vi "Write Data.vi"(8 "error in":errorcluster, 10 "Data":refnum<class "Data.lvclass">, 11 "Update Data MSG in":refnum<class "Update Controller Data MSG.lvclass">) -> (0 "error out":errorcluster, 3 "Update Data MSG out":refnum<class "Update Controller Data MSG.lvclass">)   [LabVIEW 2014]
uses:
  Update Controller Data MSG.lvclass
  reusable/Data/Data.lvclass
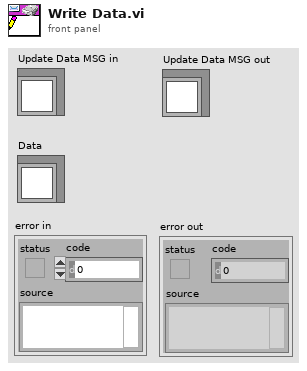
[diagram p1: front panel]
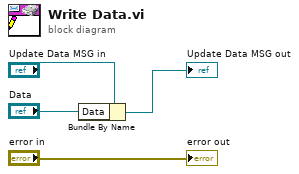
[diagram p0: block diagram]
diagram:
  n1 = Bundle By Name(cluster="Update Data MSG in", "Data"="Data") -> (→"Update Data MSG out":refnum<class "Update Controller Data MSG.lvclass">)
  "error out" <- "error in"
